vi "Send Categories to Grid.vi"(8 "error in (no error)":errorcluster, 11 "Controller in":refnum<class "Controller.lvclass">) -> (0 "error out":errorcluster, 3 "Controller out":refnum<class "Controller.lvclass">)   [LabVIEW 2024, in "Controller.lvlib" / "Controller.lvclass"]
uses:
  Controller.lvclass
  Controller.lvclass/Controller.ctl
  MC Screen/Grid Screen Messages/Populate Categories Msg/Populate Categories Msg.lvclass/Populate Categories Msg.ctl
  <vilib>/ActorFramework/Message Enqueuer/Message Enqueuer.lvclass/Message Enqueuer.ctl
  <vilib>/ActorFramework/Message Enqueuer/Enqueue.vi
  MC Screen/Grid Screen Messages/Populate Categories Msg/Populate Categories Msg.lvclass
  Applications/National Instruments/LabVIEW 2024 64-bit/vi.lib/ActorFramework/Message/Message.lvclass
  <vilib>/ActorFramework/Message Priority Queue/Priority Enqueue.vi
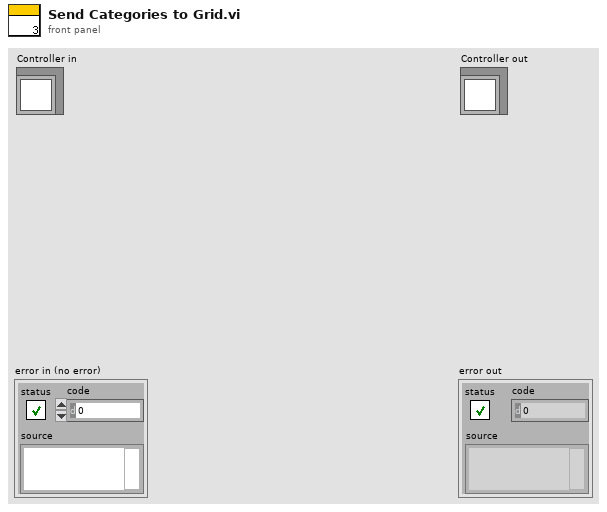
[diagram p1: front panel]
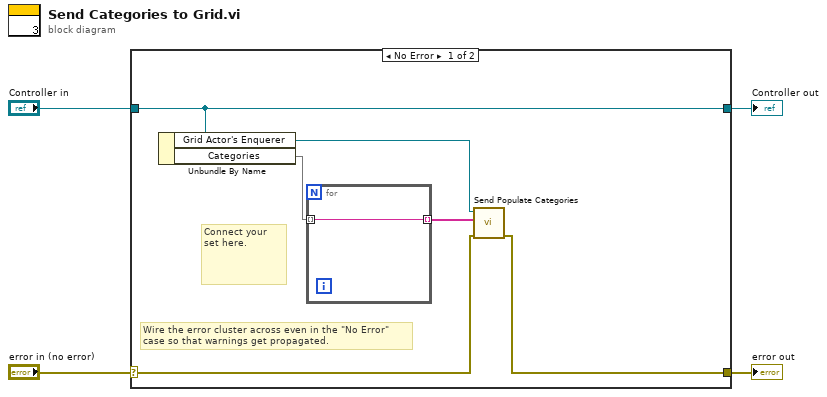
[diagram p0: block diagram]
diagram:
  n1 = case shown="No Error" "error in (no error)" {
    selector: "error in (no error)" -> [w6 w13]
    tunnel: [w5 w13] -> w3
    tunnel: [w10 w12] -> w1
    tunnel: "Controller in" -> [w10 w12]
    frame No Error {
      # "Connect your set here."
      # "Wire the error cluster across even in the \"No Error\"\ncase so that warnings get propagated."
      n2 = Unbundle By Name(w10) -> ("Grid Actor's Enquerer"=w9:refnum<class "Message Enqueuer.lvclass">, "Categories"=w8:set{string})
      n3 = for {
        tunnel: [w11] -> w7 mode=indexing
        tunnel: w8 -> [w11] mode=indexing
      }
      n4 = call "Send Populate Categories.vi"("error in (no error)"=w6, "Categories"=w7, "Message Enqueuer"=w9) -> ("error out"=w5:errorcluster)  [unwired: 7 in, 1 out]
    }
    frame Error {
    }
  }
  "error out" <- w3
  "Controller out" <- w1
